vi "RANGE Populate Configuration Data.vi"(8 "error in (no error)":errorcluster, 11 "appended path":path) -> (0 "error out":errorcluster, 2 "DAQ Data":T1={"Meter 1"={"Meter Size"=0.0, "DAQ Output (Voltage)"=0.0, "Reference (Voltage)"=0.0, "Meter Present"=FALSE, "Meter Visa"="COM3", "Gas Type"="", "SLPM Error @ Zero"=0.0, "Gas Mix Number"="", "Set STP Register"=FALSE, "Measurement Units"={"Abs. Pressure"="", "Gauge/Diff. Press."="", "Barometric Press."="", "Temperature"="", "Volume"="", "Mass"="", "Setpoint"="", "Valve Drive"="", "Totalizer"="", "Tot. Timer"="", "Tot. Avg. Flow"="", "Tot. Peak Flow"="", "Software Version"=""}}, "Meter 2"={"Meter Size"=0.0, "DAQ Output (Voltage)"=0.0, "Reference (Voltage)"=0.0, "Meter Present"=FALSE, "Meter Visa"="COM3", "Gas Type"="", "SLPM Error @ Zero"=0.0, "Gas Mix Number"="", "Set STP Register"=FALSE, "Measurement Units"={"Abs. Pressure"="", "Gauge/Diff. Press."="", "Barometric Press."="", "Temperature"="", "Volume"="", "Mass"="", "Setpoint"="", "Valve Drive"="", "Totalizer"="", "Tot. Timer"="", "Tot. Avg. Flow"="", "Tot. Peak Flow"="", "Software Version"=""}}, "Meter 3"={"Meter Size"=0.0, "DAQ Output (Voltage)"=0.0, "Reference (Voltage)"=0.0, "Meter Present"=FALSE, "Meter Visa"="COM3", "Gas Type"="", "SLPM Error @ Zero"=0.0, "Gas Mix Number"="", "Set STP Register"=FALSE, "Measurement Units"={"Abs. Pressure"="", "Gauge/Diff. Press."="", "Barometric Press."="", "Temperature"="", "Volume"="", "Mass"="", "Setpoint"="", "Valve Drive"="", "Totalizer"="", "Tot. Timer"="", "Tot. Avg. Flow"="", "Tot. Peak Flow"="", "Software Version"=""}}, "Meter 4"={"Meter Size"=0.0, "DAQ Output (Voltage)"=0.0, "Reference (Voltage)"=0.0, "Meter Present"=FALSE, "Meter Visa"="COM3", "Gas Type"="", "SLPM Error @ Zero"=0.0, "Gas Mix Number"="", "Set STP Register"=FALSE, "Measurement Units"={"Abs. Pressure"="", "Gauge/Diff. Press."="", "Barometric Press."="", "Temperature"="", "Volume"="", "Mass"="", "Setpoint"="", "Valve Drive"="", "Totalizer"="", "Tot. Timer"="", "Tot. Avg. Flow"="", "Tot. Peak Flow"="", "Software Version"=""}}, "Meter 5"={"Meter Size"=0.0, "DAQ Output (Voltage)"=0.0, "Reference (Voltage)"=0.0, "Meter Present"=FALSE, "Meter Visa"="COM3", "Gas Type"="", "SLPM Error @ Zero"=0.0, "Gas Mix Number"="", "Set STP Register"=FALSE, "Measurement Units"={"Abs. Pressure"="", "Gauge/Diff. Press."="", "Barometric Press."="", "Temperature"="", "Volume"="", "Mass"="", "Setpoint"="", "Valve Drive"="", "Totalizer"="", "Tot. Timer"="", "Tot. Avg. Flow"="", "Tot. Peak Flow"="", "Software Version"=""}}, "Meter 6"={"Meter Size"=0.0, "DAQ Output (Voltage)"=0.0, "Reference (Voltage)"=0.0, "Meter Present"=FALSE, "Meter Visa"="COM3", "Gas Type"="", "SLPM Error @ Zero"=0.0, "Gas Mix Number"="", "Set STP Register"=FALSE, "Measurement Units"={"Abs. Pressure"="", "Gauge/Diff. Press."="", "Barometric Press."="", "Temperature"="", "Volume"="", "Mass"="", "Setpoint"="", "Valve Drive"="", "Totalizer"="", "Tot. Timer"="", "Tot. Avg. Flow"="", "Tot. Peak Flow"="", "Software Version"=""}}, "Meter Bank 1"={"Flow Rate (BTU/HR)"=0.0, "ANSI Placeholder Array"=[], "15 Sec Avg Array"=[], "30 Sec Avg Array "=[], "ANSI Average (BTU/HR)"=0.0, "Panel Data"={"Meter Type (Gas)"="", "Heating Value (BTU/ft³)"=0.0, "Ft³ / Hr (SCFH)"=0.0, "15 Second Average (BTU/HR)"=0.0, "30 Second Average (BTU/HR)"=0.0, "Mass Flow"=0.0, "Vol. Flow"=0.0, "Gas Temperature"=0.0, "Gas Pressure"=0.0, "Tot.Flow"=0.0}, "Start ANSI"=FALSE, "ANSI Start Time"=0.0, "Restart ANSI"=FALSE, "Meter ID"=""}, "Meter Bank 2"={"Flow Rate (BTU/HR)"=0.0, "ANSI Placeholder Array"=[], "15 Sec Avg Array"=[], "30 Sec Avg Array "=[], "ANSI Average (BTU/HR)"=0.0, "Panel Data"={"Meter Type (Gas)"="", "Heating Value (BTU/ft³)"=0.0, "Ft³ / Hr (SCFH)"=0.0, "15 Second Average (BTU/HR)"=0.0, "30 Second Average (BTU/HR)"=0.0, "Mass Flow"=0.0, "Vol. Flow"=0.0, "Gas Temperature"=0.0, "Gas Pressure"=0.0, "Tot.Flow"=0.0}, "Start ANSI"=FALSE, "ANSI Start Time"=0.0, "Restart ANSI"=FALSE, "Meter ID"=""}, "Meter Bank 3"={"Flow Rate (BTU/HR)"=0.0, "ANSI Placeholder Array"=[], "15 Sec Avg Array"=[], "30 Sec Avg Array "=[], "ANSI Average (BTU/HR)"=0.0, "Panel Data"={"Meter Type (Gas)"="", "Heating Value (BTU/ft³)"=0.0, "Ft³ / Hr (SCFH)"=0.0, "15 Second Average (BTU/HR)"=0.0, "30 Second Average (BTU/HR)"=0.0, "Mass Flow"=0.0, "Vol. Flow"=0.0, "Gas Temperature"=0.0, "Gas Pressure"=0.0, "Tot.Flow"=0.0}, "Start ANSI"=FALSE, "ANSI Start Time"=0.0, "Restart ANSI"=FALSE, "Meter ID"=""}, "Threshold Voltage (NI DAQ)"=0.0, "Use RS232 Data Collection"=FALSE, "Use Auto Switching"=FALSE}, 3 "all rows":string[][](array[string]))   [LabVIEW 2018]
uses:
  Type Definitions/RANGE DAQ Data Four Meters.ctl
  Type Definitions/RANGE DAQ Data.ctl
  Drivers/Omega FMA-1600A Series Gas Flow Meter/Type Definitions/FMA1600A Gas Type.ctl
  Drivers/Omega FMA-1600A Series Gas Flow Meter/Type Definitions/FMA1600A Units String.ctl
  Type Definitions/RANGE GAS Data.ctl
  Type Definitions/RANGE Panel Data.ctl
  <vilib>/Utility/file.llb/Read From Spreadsheet File (string).vi
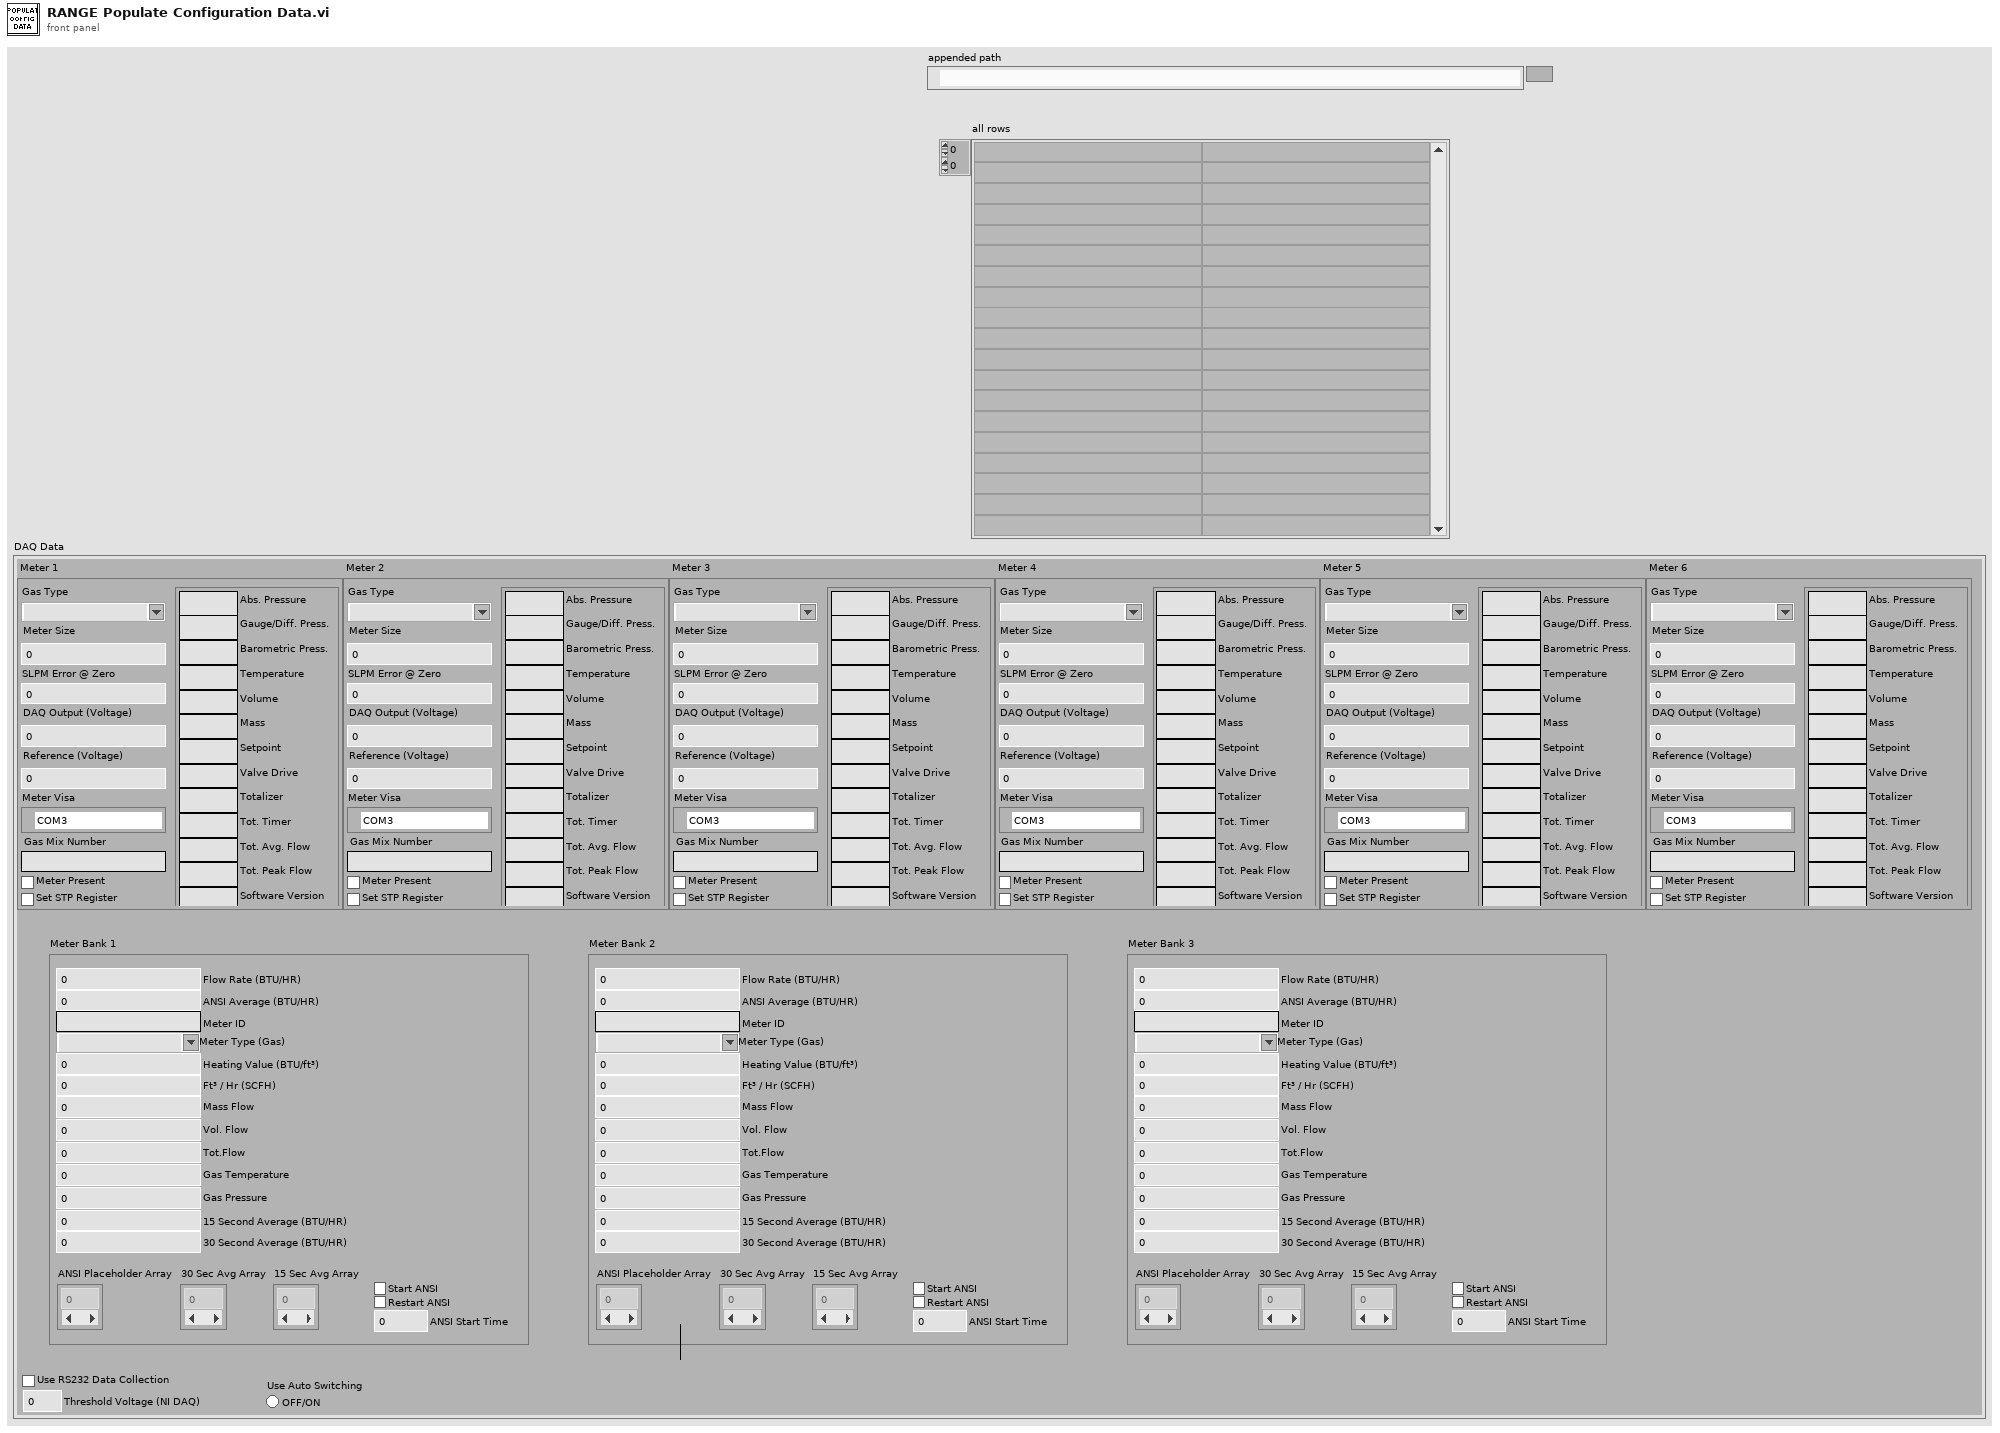
[diagram p1: front panel]
types:
  T1 = typedef "RANGE DAQ Data Four Meters.ctl" = cluster{"Meter 1":T2, "Meter 2":T2, "Meter 3":T2, "Meter 4":T2, "Meter 5":T2, "Meter 6":T2, "Meter Bank 1":T5, "Meter Bank 2":T5, "Meter Bank 3":T5, "Threshold Voltage (NI DAQ)":dbl, "Use RS232 Data Collection":bool, "Use Auto Switching":bool}
  T2 = typedef "RANGE DAQ Data.ctl" = cluster{"Meter Size":dbl, "DAQ Output (Voltage)":dbl, "Reference (Voltage)":dbl, "Meter Present":bool, "Meter Visa":refnum<visa-resource-name>, "Gas Type":T3, "SLPM Error @ Zero":dbl, "Gas Mix Number":string, "Set STP Register":bool, "Measurement Units":T4}
  T3 = typedef "FMA1600A Gas Type.ctl" = string
  T4 = typedef "FMA1600A Units String.ctl" = cluster{"Abs. Pressure":string, "Gauge/Diff. Press.":string, "Barometric Press.":string, "Temperature":string, "Volume":string, "Mass":string, "Setpoint":string, "Valve Drive":string, "Totalizer":string, "Tot. Timer":string, "Tot. Avg. Flow":string, "Tot. Peak Flow":string, "Software Version":string}
  T5 = typedef "RANGE GAS Data.ctl" = cluster{"Flow Rate (BTU/HR)":dbl, "ANSI Placeholder Array":dbl[], "15 Sec Avg Array":dbl[], "30 Sec Avg Array ":dbl[], "ANSI Average (BTU/HR)":dbl, "Panel Data":T6, "Start ANSI":bool, "ANSI Start Time":dbl, "Restart ANSI":bool, "Meter ID":string}
  T6 = typedef "RANGE Panel Data.ctl" = cluster{"Meter Type (Gas)":T3, "Heating Value (BTU/ft³)":dbl, "Ft³ / Hr (SCFH)":dbl, "15 Second Average (BTU/HR)":dbl, "30 Second Average (BTU/HR)":dbl, "Mass Flow":dbl, "Vol. Flow":dbl, "Gas Temperature":dbl, "Gas Pressure":dbl, "Tot.Flow":dbl}
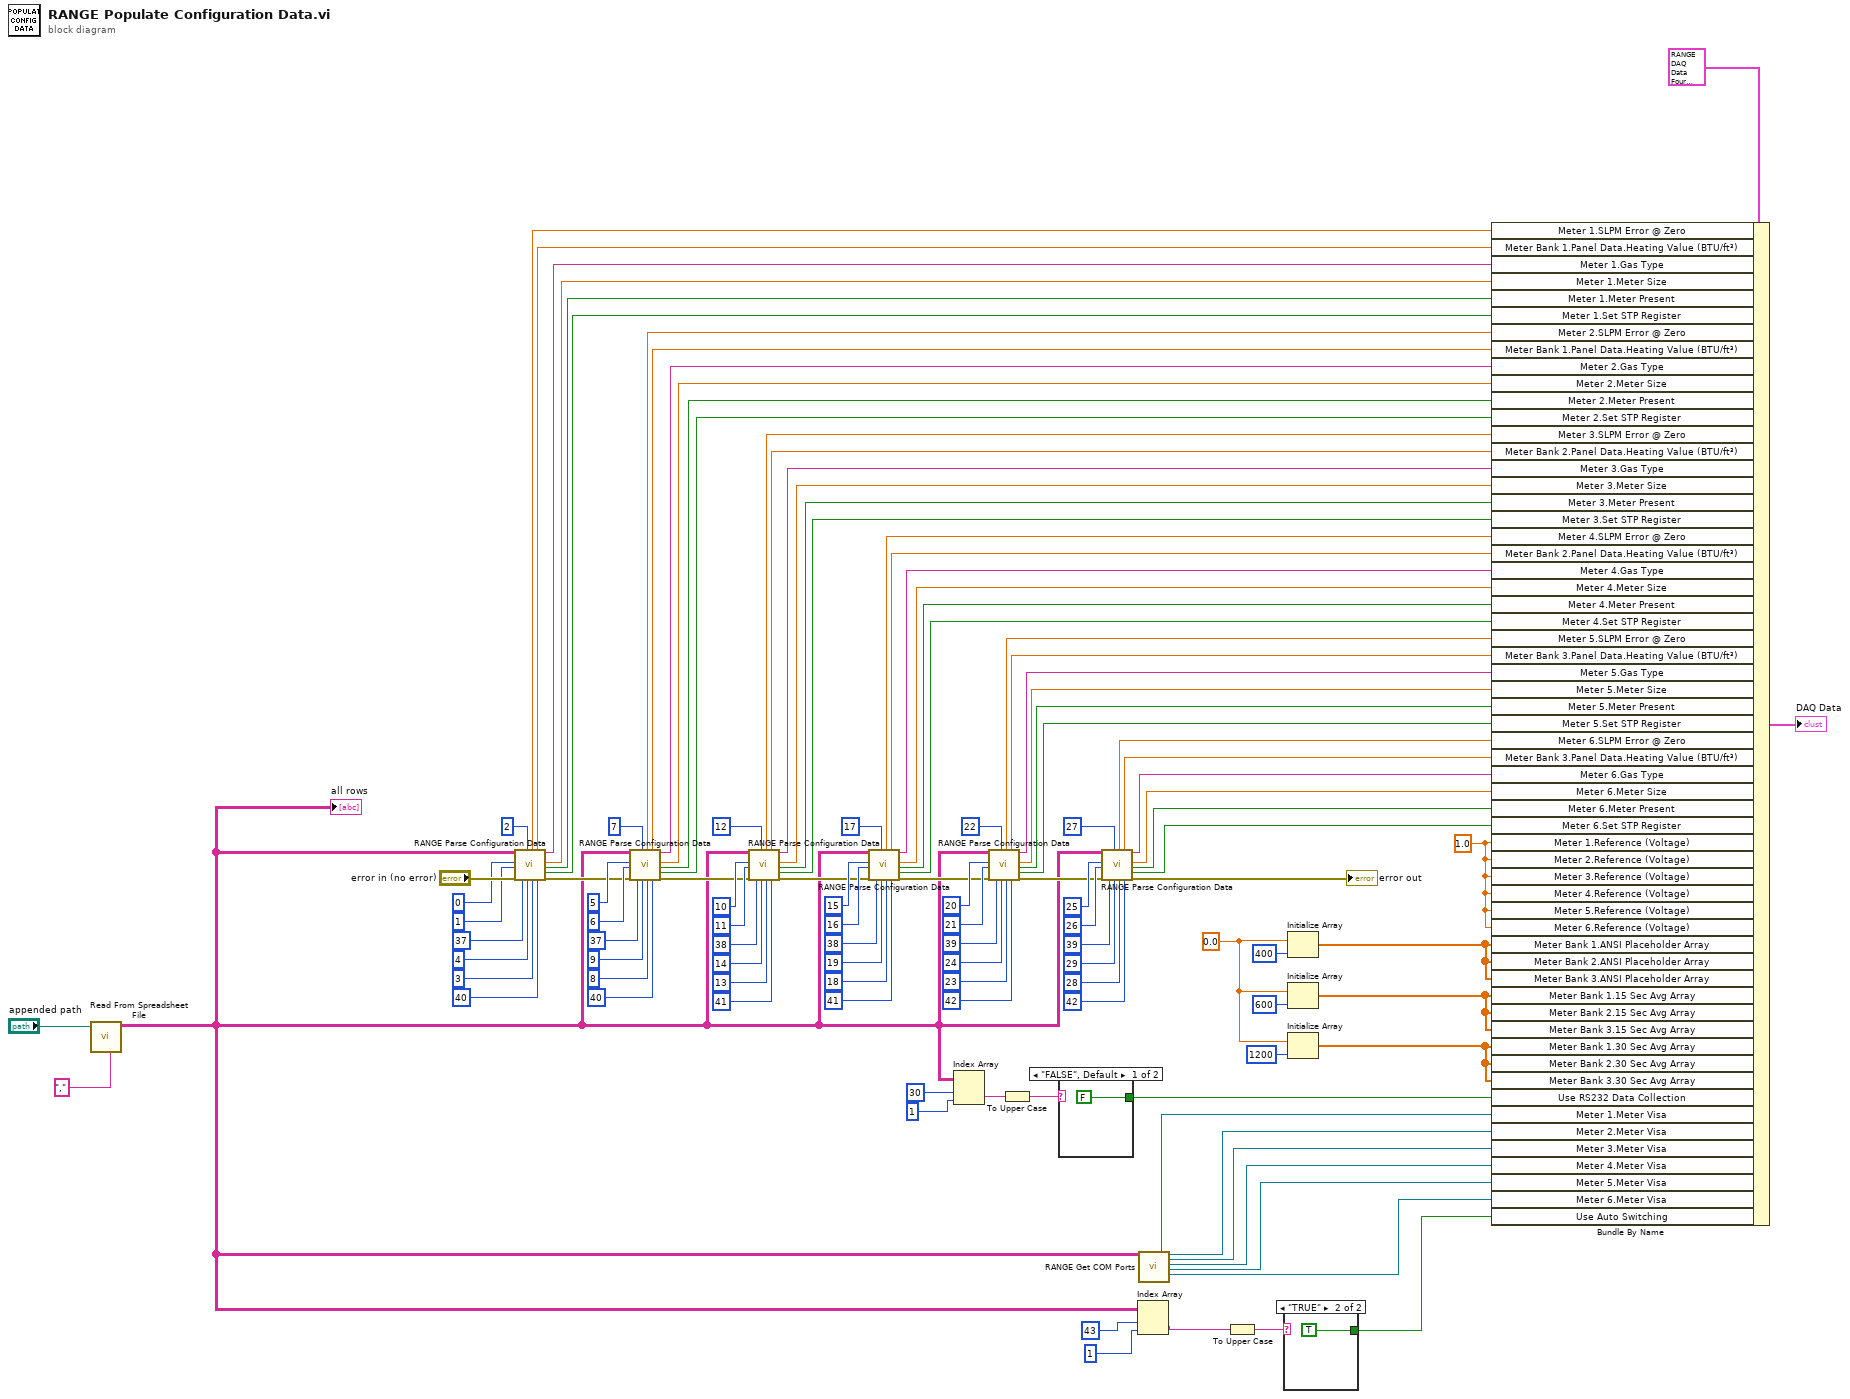
[diagram p0: block diagram]
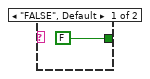
[diagram p2: hidden frame]
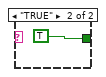
[diagram p3: hidden frame]
diagram:
  w106 = 0.0
  w101 = 1.0
  n1 = call-poly <vilib>:"Read From Spreadsheet File.vi"("delimiter (\\t)"="," ("delimiter (\\t)"), "file path (dialog if empty)"="appended path") -> ("all rows"=w6:string[][])  [unwired: 5 in, 4 out]
  "all rows" <- w6
  n2 = call "RANGE Parse Configuration Data.vi"("all rows"=w6, "Meter Type Index"=0 ("disabled index (row)"), "Meter Size Index"=1 ("disabled index (col)"), "Error In"="error in (no error)", "Heating Value Index"=37 ("Natural Gas Heating Value Index"), "Accuracy Reading Index"=2 ("disabled index (row)"), "Meter Present Index"=4, "Accuracy Full Scale Index"=3, "Set STP Register"=40) -> ("SLPM Error @ Zero"=w43:dbl, "Heating Value (BTU/ft³)"=w31:dbl, "Meter Type (Gas)"=w60:T3, "Meter Size"=w61:dbl, "Meter Present"=w62:bool, "STP Register Set"=w12:bool, "Error Out"=w79:errorcluster)  [unwired: 4 in]
  n3 = call "RANGE Parse Configuration Data.vi"("all rows"=w6, "Meter Type Index"=5 ("disabled index (row)"), "Meter Size Index"=6 ("disabled index (row)"), "Error In"=w79, "Heating Value Index"=37 ("Natural Gas Heating Value Index"), "Accuracy Reading Index"=7, "Meter Present Index"=9 ("disabled index (row)"), "Accuracy Full Scale Index"=8, "Set STP Register"=40) -> ("SLPM Error @ Zero"=w42:dbl, "Heating Value (BTU/ft³)"=w30:dbl, "Meter Type (Gas)"=w64:T3, "Meter Size"=w65:dbl, "Meter Present"=w66:bool, "STP Register Set"=w11:bool, "Error Out"=w80:errorcluster)  [unwired: 4 in]
  n4 = call "RANGE Parse Configuration Data.vi"("all rows"=w6, "Meter Type Index"=10 ("disabled index (row)"), "Meter Size Index"=11 ("disabled index (row)"), "Error In"=w80, "Heating Value Index"=38 ("Natural Gas Heating Value Index"), "Accuracy Reading Index"=12, "Meter Present Index"=14 ("disabled index (row)"), "Accuracy Full Scale Index"=13, "Set STP Register"=41) -> ("SLPM Error @ Zero"=w41:dbl, "Heating Value (BTU/ft³)"=w29:dbl, "Meter Type (Gas)"=w67:T3, "Meter Size"=w68:dbl, "Meter Present"=w69:bool, "STP Register Set"=w10:bool, "Error Out"=w81:errorcluster)  [unwired: 4 in]
  n5 = call "RANGE Parse Configuration Data.vi"("all rows"=w6, "Meter Type Index"=15 ("disabled index (row)"), "Meter Size Index"=16 ("disabled index (row)"), "Error In"=w81, "Heating Value Index"=38 ("Natural Gas Heating Value Index"), "Accuracy Reading Index"=17, "Meter Present Index"=19 ("disabled index (row)"), "Accuracy Full Scale Index"=18, "Set STP Register"=41) -> ("SLPM Error @ Zero"=w40:dbl, "Heating Value (BTU/ft³)"=w28:dbl, "Meter Type (Gas)"=w70:T3, "Meter Size"=w71:dbl, "Meter Present"=w72:bool, "STP Register Set"=w9:bool, "Error Out"=w82:errorcluster)  [unwired: 4 in]
  n6 = Index Array(array=w6, index (row)=30, index (col)=1 ("disabled index (col)")) -> (element=w112:string)
  n7 = call "RANGE Parse Configuration Data.vi"("all rows"=w6, "Meter Type Index"=20 ("disabled index (row)"), "Meter Size Index"=21 ("disabled index (row)"), "Error In"=w82, "Heating Value Index"=39 ("Natural Gas Heating Value Index"), "Accuracy Reading Index"=22, "Meter Present Index"=24 ("disabled index (row)"), "Accuracy Full Scale Index"=23, "Set STP Register"=42) -> ("SLPM Error @ Zero"=w39:dbl, "Heating Value (BTU/ft³)"=w27:dbl, "Meter Type (Gas)"=w73:T3, "Meter Size"=w74:dbl, "Meter Present"=w75:bool, "STP Register Set"=w8:bool, "Error Out"=w83:errorcluster)  [unwired: 4 in]
  n8 = To Upper Case(1:w112) -> (0:w113:string)
  n9 = case shown="\"FALSE\", Default" w113 {
    tunnel: [FALSE TRUE] -> w114
    frame "FALSE", Default {
    }
    frame "TRUE" {
    }
  }
  n10 = call "RANGE Parse Configuration Data.vi"("all rows"=w6, "Meter Type Index"=25 ("disabled index (row)"), "Meter Size Index"=26 ("disabled index (row)"), "Error In"=w83, "Heating Value Index"=39 ("Natural Gas Heating Value Index"), "Accuracy Reading Index"=27, "Meter Present Index"=29 ("disabled index (row)"), "Accuracy Full Scale Index"=28, "Set STP Register"=42) -> ("SLPM Error @ Zero"=w38:dbl, "Heating Value (BTU/ft³)"=w26:dbl, "Meter Type (Gas)"=w76:T3, "Meter Size"=w77:dbl, "Meter Present"=w78:bool, "STP Register Set"=w7:bool, "Error Out"=→"error out":errorcluster)  [unwired: 4 in]
  n11 = Index Array(array=w6, index (row)=43 ("disabled index (row)"), index (col)=1 ("disabled index (col)")) -> (element=w2:string)
  n12 = call "RANGE Get COM Ports.vi"("all rows"=w6) -> ("Meter 1"=w37:refnum<visa-resource-name>, "Meter 2"=w36:refnum<visa-resource-name>, "Meter 3"=w35:refnum<visa-resource-name>, "Meter 4"=w34:refnum<visa-resource-name>, "Meter 5"=w33:refnum<visa-resource-name>, "Meter 6"=w32:refnum<visa-resource-name>)  [unwired: 12 in, 1 out]
  n13 = To Upper Case(1:w2) -> (0:w3:string)
  n14 = case shown="\"TRUE\"" w3 {
    tunnel: [FALSE TRUE] -> w1
    frame "FALSE", Default {
    }
    frame "TRUE" {
    }
  }
  n15 = Initialize Array(w106, 400) -> (w103:dbl[])
  n16 = Initialize Array(w106, 600) -> (w107:dbl[])
  n17 = Initialize Array(w106, 1200) -> (w108:dbl[])
  n18 = Bundle By Name(cluster=T1 {"Meter 1"={"Meter Size"=0.0, "DAQ Output (Voltage)"=0.0, "Reference (Voltage)"=0.0, "Meter Present"=FALSE, "Meter Visa"="COM3", "Gas Type"="", "SLPM Error @ Zero"=0.0, "Gas Mix Number"="", "Set STP Register"=FALSE, "Measurement Units"={"Abs. Pressure"="", "Gauge/Diff. Press."="", "Barometric Press."="", "Temperature"="", "Volume"="", "Mass"="", "Setpoint"="", "Valve Drive"="", "Totalizer"="", "Tot. Timer"="", "Tot. Avg. Flow"="", "Tot. Peak Flow"="", "Software Version"=""}}, "Meter 2"={"Meter Size"=0.0, "DAQ Output (Voltage)"=0.0, "Reference (Voltage)"=0.0, "Meter Present"=FALSE, "Meter Visa"="COM3", "Gas Type"="", "SLPM Error @ Zero"=0.0, "Gas Mix Number"="", "Set STP Register"=FALSE, "Measurement Units"={"Abs. Pressure"="", "Gauge/Diff. Press."="", "Barometric Press."="", "Temperature"="", "Volume"="", "Mass"="", "Setpoint"="", "Valve Drive"="", "Totalizer"="", "Tot. Timer"="", "Tot. Avg. Flow"="", "Tot. Peak Flow"="", "Software Version"=""}}, "Meter 3"={"Meter Size"=0.0, "DAQ Output (Voltage)"=0.0, "Reference (Voltage)"=0.0, "Meter Present"=FALSE, "Meter Visa"="COM3", "Gas Type"="", "SLPM Error @ Zero"=0.0, "Gas Mix Number"="", "Set STP Register"=FALSE, "Measurement Units"={"Abs. Pressure"="", "Gauge/Diff. Press."="", "Barometric Press."="", "Temperature"="", "Volume"="", "Mass"="", "Setpoint"="", "Valve Drive"="", "Totalizer"="", "Tot. Timer"="", "Tot. Avg. Flow"="", "Tot. Peak Flow"="", "Software Version"=""}}, "Meter 4"={"Meter Size"=0.0, "DAQ Output (Voltage)"=0.0, "Reference (Voltage)"=0.0, "Meter Present"=FALSE, "Meter Visa"="COM3", "Gas Type"="", "SLPM Error @ Zero"=0.0, "Gas Mix Number"="", "Set STP Register"=FALSE, "Measurement Units"={"Abs. Pressure"="", "Gauge/Diff. Press."="", "Barometric Press."="", "Temperature"="", "Volume"="", "Mass"="", "Setpoint"="", "Valve Drive"="", "Totalizer"="", "Tot. Timer"="", "Tot. Avg. Flow"="", "Tot. Peak Flow"="", "Software Version"=""}}, "Meter 5"={"Meter Size"=0.0, "DAQ Output (Voltage)"=0.0, "Reference (Voltage)"=0.0, "Meter Present"=FALSE, "Meter Visa"="COM3", "Gas Type"="", "SLPM Error @ Zero"=0.0, "Gas Mix Number"="", "Set STP Register"=FALSE, "Measurement Units"={"Abs. Pressure"="", "Gauge/Diff. Press."="", "Barometric Press."="", "Temperature"="", "Volume"="", "Mass"="", "Setpoint"="", "Valve Drive"="", "Totalizer"="", "Tot. Timer"="", "Tot. Avg. Flow"="", "Tot. Peak Flow"="", "Software Version"=""}}, "Meter 6"={"Meter Size"=0.0, "DAQ Output (Voltage)"=0.0, "Reference (Voltage)"=0.0, "Meter Present"=FALSE, "Meter Visa"="COM3", "Gas Type"="", "SLPM Error @ Zero"=0.0, "Gas Mix Number"="", "Set STP Register"=FALSE, "Measurement Units"={"Abs. Pressure"="", "Gauge/Diff. Press."="", "Barometric Press."="", "Temperature"="", "Volume"="", "Mass"="", "Setpoint"="", "Valve Drive"="", "Totalizer"="", "Tot. Timer"="", "Tot. Avg. Flow"="", "Tot. Peak Flow"="", "Software Version"=""}}, "Meter Bank 1"={"Flow Rate (BTU/HR)"=0.0, "ANSI Placeholder Array"=[], "15 Sec Avg Array"=[], "30 Sec Avg Array "=[], "ANSI Average (BTU/HR)"=0.0, "Panel Data"={"Meter Type (Gas)"="", "Heating Value (BTU/ft³)"=0.0, "Ft³ / Hr (SCFH)"=0.0, "15 Second Average (BTU/HR)"=0.0, "30 Second Average (BTU/HR)"=0.0, "Mass Flow"=0.0, "Vol. Flow"=0.0, "Gas Temperature"=0.0, "Gas Pressure"=0.0, "Tot.Flow"=0.0}, "Start ANSI"=FALSE, "ANSI Start Time"=0.0, "Restart ANSI"=FALSE, "Meter ID"=""}, "Meter Bank 2"={"Flow Rate (BTU/HR)"=0.0, "ANSI Placeholder Array"=[], "15 Sec Avg Array"=[], "30 Sec Avg Array "=[], "ANSI Average (BTU/HR)"=0.0, "Panel Data"={"Meter Type (Gas)"="", "Heating Value (BTU/ft³)"=0.0, "Ft³ / Hr (SCFH)"=0.0, "15 Second Average (BTU/HR)"=0.0, "30 Second Average (BTU/HR)"=0.0, "Mass Flow"=0.0, "Vol. Flow"=0.0, "Gas Temperature"=0.0, "Gas Pressure"=0.0, "Tot.Flow"=0.0}, "Start ANSI"=FALSE, "ANSI Start Time"=0.0, "Restart ANSI"=FALSE, "Meter ID"=""}, "Meter Bank 3"={"Flow Rate (BTU/HR)"=0.0, "ANSI Placeholder Array"=[], "15 Sec Avg Array"=[], "30 Sec Avg Array "=[], "ANSI Average (BTU/HR)"=0.0, "Panel Data"={"Meter Type (Gas)"="", "Heating Value (BTU/ft³)"=0.0, "Ft³ / Hr (SCFH)"=0.0, "15 Second Average (BTU/HR)"=0.0, "30 Second Average (BTU/HR)"=0.0, "Mass Flow"=0.0, "Vol. Flow"=0.0, "Gas Temperature"=0.0, "Gas Pressure"=0.0, "Tot.Flow"=0.0}, "Start ANSI"=FALSE, "ANSI Start Time"=0.0, "Restart ANSI"=FALSE, "Meter ID"=""}, "Threshold Voltage (NI DAQ)"=0.2, "Use RS232 Data Collection"=FALSE, "Use Auto Switching"=FALSE} ("DAQ Data"), "Meter 1.SLPM Error @ Zero"=w43, "Meter Bank 1.Panel Data.Heating Value (BTU/ft³)"=w31, "Meter 1.Gas Type"=w60, "Meter 1.Meter Size"=w61, "Meter 1.Meter Present"=w62, "Meter 1.Set STP Register"=w12, "Meter 2.SLPM Error @ Zero"=w42, "Meter Bank 1.Panel Data.Heating Value (BTU/ft³)"=w30, "Meter 2.Gas Type"=w64, "Meter 2.Meter Size"=w65, "Meter 2.Meter Present"=w66, "Meter 2.Set STP Register"=w11, "Meter 3.SLPM Error @ Zero"=w41, "Meter Bank 2.Panel Data.Heating Value (BTU/ft³)"=w29, "Meter 3.Gas Type"=w67, "Meter 3.Meter Size"=w68, "Meter 3.Meter Present"=w69, "Meter 3.Set STP Register"=w10, "Meter 4.SLPM Error @ Zero"=w40, "Meter Bank 2.Panel Data.Heating Value (BTU/ft³)"=w28, "Meter 4.Gas Type"=w70, "Meter 4.Meter Size"=w71, "Meter 4.Meter Present"=w72, "Meter 4.Set STP Register"=w9, "Meter 5.SLPM Error @ Zero"=w39, "Meter Bank 3.Panel Data.Heating Value (BTU/ft³)"=w27, "Meter 5.Gas Type"=w73, "Meter 5.Meter Size"=w74, "Meter 5.Meter Present"=w75, "Meter 5.Set STP Register"=w8, "Meter 6.SLPM Error @ Zero"=w38, "Meter Bank 3.Panel Data.Heating Value (BTU/ft³)"=w26, "Meter 6.Gas Type"=w76, "Meter 6.Meter Size"=w77, "Meter 6.Meter Present"=w78, "Meter 6.Set STP Register"=w7, "Meter 1.Reference (Voltage)"=w101, "Meter 2.Reference (Voltage)"=w101, "Meter 3.Reference (Voltage)"=w101, "Meter 4.Reference (Voltage)"=w101, "Meter 5.Reference (Voltage)"=w101, "Meter 6.Reference (Voltage)"=w101, "Meter Bank 1.ANSI Placeholder Array"=w103, "Meter Bank 2.ANSI Placeholder Array"=w103, "Meter Bank 3.ANSI Placeholder Array"=w103, "Meter Bank 1.15 Sec Avg Array"=w107, "Meter Bank 2.15 Sec Avg Array"=w107, "Meter Bank 3.15 Sec Avg Array"=w107, "Meter Bank 1.30 Sec Avg Array"=w108, "Meter Bank 2.30 Sec Avg Array"=w108, "Meter Bank 3.30 Sec Avg Array"=w108, "Use RS232 Data Collection"=w114, "Meter 1.Meter Visa"=w37, "Meter 2.Meter Visa"=w36, "Meter 3.Meter Visa"=w35, "Meter 4.Meter Visa"=w34, "Meter 5.Meter Visa"=w33, "Meter 6.Meter Visa"=w32, "Use Auto Switching"=w1) -> (→"DAQ Data":T1)
